vi "Step to JSON String.vi"(8 "error in (no error)":errorcluster, 11 "Base Step in":refnum<class "Base Step.lvclass">) -> (0 "error out":errorcluster, 2 "Config String":string, 3 "Base Step out":refnum<class "Base Step.lvclass">)   [LabVIEW 2024, in "Ramses Sequencer.lvlib" / "Base Step.lvclass"]
uses:
  Base Step.lvclass
  <vilib>/Utility/Data Type/Type Definitions/Data Type.ctl
  Base Step.lvclass/Base Step.ctl
  e2cf0667-7960-454c-8904-34309a959e26.vi
  <vilib>/JDP Science/JSONtext/LVClass Serializer/JSONtext LVClass Serializer.lvclass
  <vilib>/JDP Science/JSONtext/JSONtext.lvlib
  <vilib>/Utility/Data Type/NI_Data Type.lvlib
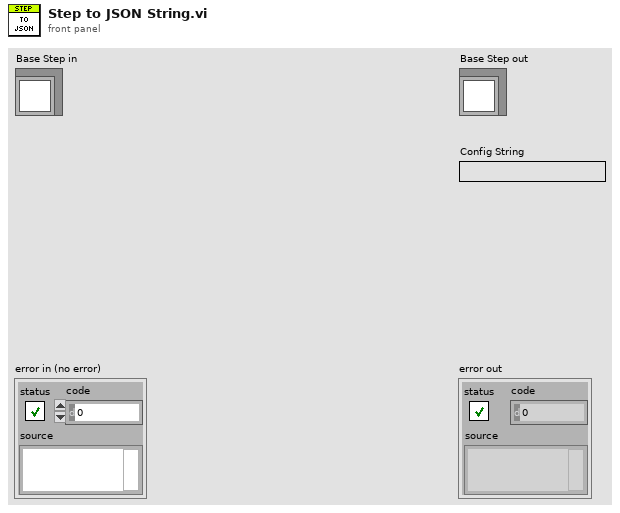
[diagram p1: front panel]
types:
  T1 = typedef "NI_Data Type.lvlib/Data Type.ctl" = enum8{"Invalid Type", "Void", "I8", "I16", "I32", "I64", "U8", "U16", "U32", "U64", "Single Float", "Double Float", "Extended Float", "Single Complex", "Double Complex", "Extended Complex", "Enum U8", "Enum U16", "Enum U32", "Enum U64", "Single Float With Unit", "Double Float With Unit", "Extended Float With Unit", "Single Complex with Unit", "Double Complex with Unit", "Extended Complex with Unit", "Boolean", "String", "Path", "Picture", "Tag", "Array", "Cluster", "Variant", "LV Variant", "Waveform", "Timestamp", "Digital Waveform", "Digital Data", "ExpressData", "Refnum", "External Data", "VI", "Poly VI", "LabVIEW Class Instance", "Fixed Point", "Set Collection", "Map Collection"}
  T2 = cluster{"Class Name":string, "Name":string, "Properties":cluster{string, "type":T1, "<JSON>":string}[]}
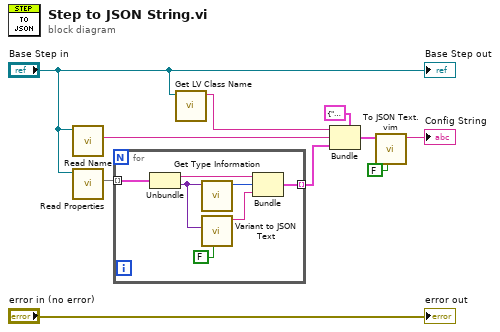
[diagram p0: block diagram]
diagram:
  n1 = call-dynamic "Read Name.vi"("Base Step in"="Base Step in") -> ("Name"=w8:string)  [unwired: 8 in, 2 out]
  n2 = call "Read Properties.vi"("Base Step in"="Base Step in") -> ("Properties"=w9:map{string, variant})  [unwired: 8 in, 2 out]
  n3 = for {
    tunnel: w9 -> [w17] mode=indexing
    tunnel: [w15] -> w1 mode=indexing
    n4 = Unbundle(w17) -> (w16:string, "Data"=w12:variant)
    n5 = call <vilib>:"Get Type Information.vi"("variant"=w12) -> ("type"=w11:T1)  [unwired: 6 in, 4 out]
    n6 = call <vilib>:"Variant to JSON Text.vi"("Pretty Print?"=FALSE, "Variant"=w12) -> ("<JSON>"=w13:string)  [unwired: 7 in, 2 out]
    n7 = Bundle(w16, "type"=w11, "<JSON>"=w13) -> (w15:cluster{string, "type":T1, "<JSON>":string})  [unwired: 1 in]
  }
  n8 = call <vilib>:"Get LV Class Name.vi"("object"="Base Step in") -> ("class name"=w3:string)  [unwired: 9 in, 1 out]
  n9 = Bundle(cluster=T2 {"Class Name"="", "Name"="", "Properties"=[]}, "Class Name"=w3, "Name"=w8, "Properties"=w1) -> (w7:T2)
  n10 = call "To JSON Text.vim"("Pretty Print?"=FALSE, "Anything"=w7) -> ("<JSON>"=→"Config String":string)  [unwired: 8 in, 1 out]
  "error out" <- "error in (no error)"
  "Base Step out" <- "Base Step in"
